vi "Parse Value.vi"(8 "error in (no error)":errorcluster, 11 "Alpaca CLI Parser in":refnum<class "JSON Parser.lvclass">) -> (0 "error out":errorcluster, 2 "Value":variant, 3 "Alpaca CLI Parser out":refnum<class "JSON Parser.lvclass">)   [LabVIEW 2019, in "JKI JSON Serialization.lvlib" / "JSON Parser.lvclass"]
doc: "JKI JSON 1.1.10.37\nTomi Maila - JKI\nCopyright (c) 2017, JKI"
uses:
  JSON Parser.lvclass
  C:/Users/Patrick/Documents/GitHub/Instrument-Framework/lvsrc/SMOs/JSON-RPC-2019/lv-venv/lv.lib/vi.lib/addons/_JKI.lib/Serialization/JSON/Deserializer/Parser/Parser.lvclass
  Parser/Parser.lvclass/Parser.ctl
  JSON Lexer/JSON Token Type.ctl
  Parser/Lookahead.vi
  JSON Lexer/JSON Lexer.lvclass
  JKI JSON Serialization.lvlib
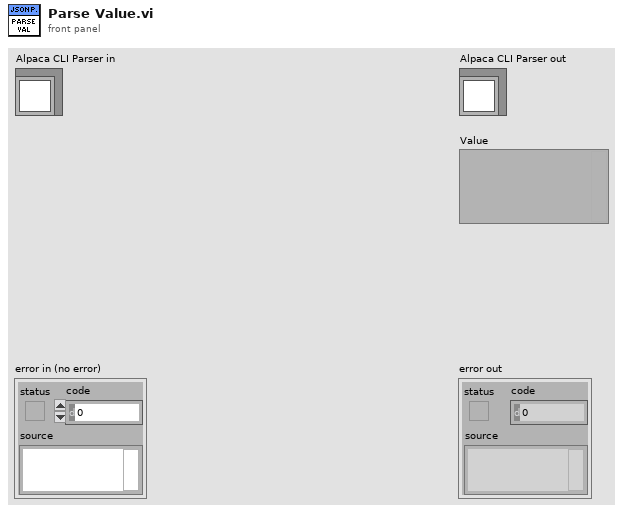
[diagram p1: front panel]
types:
  T1 = typedef "JKI JSON Serialization.lvlib/JSON Lexer.lvclass/JSON Token Type.ctl" = enum32{"unknown", "comma", "end-label", "begin-object", "end-object", "begin-array", "end-array", "quoted-string", "boolean", "exponential-number", "decimal-number", "integer-number", "special-number", "null", "symbol", "whitespace", "EOF"}
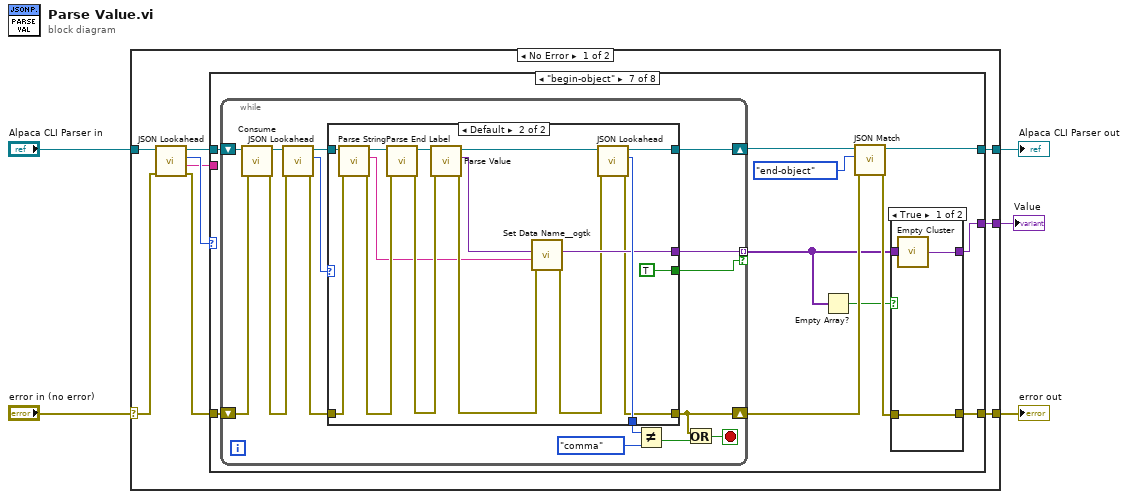
[diagram p0: block diagram]
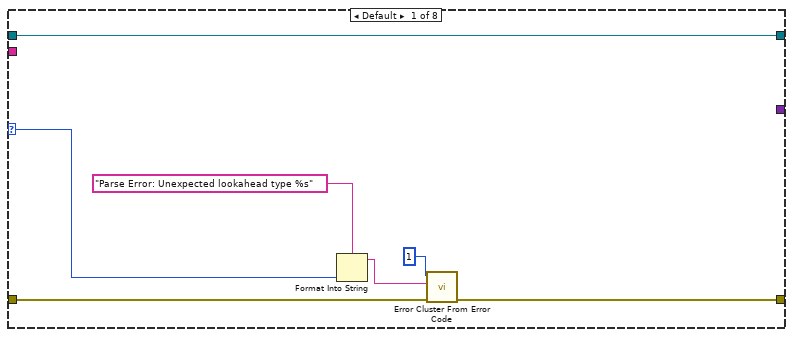
[diagram p2: hidden frame]
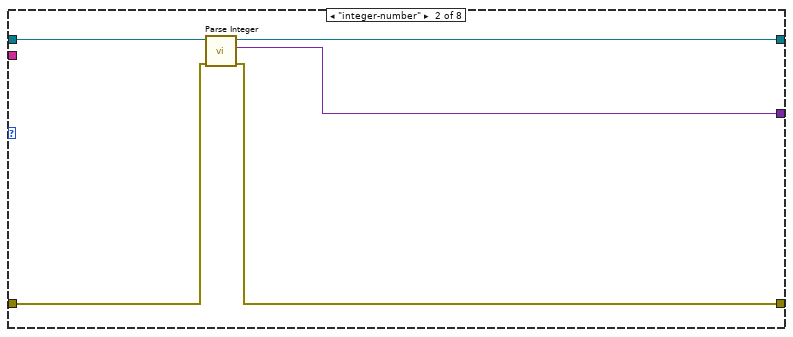
[diagram p3: hidden frame]
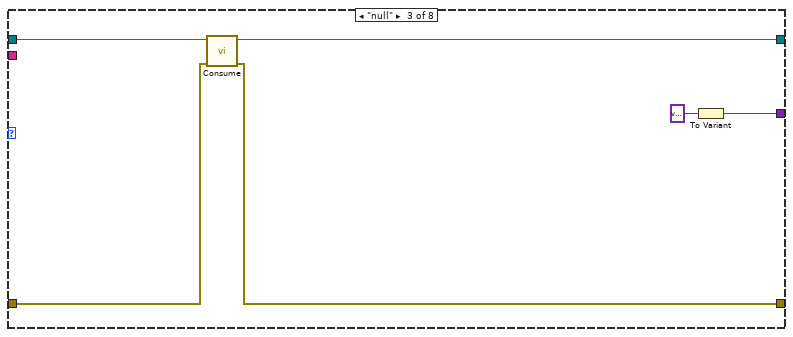
[diagram p4: hidden frame]
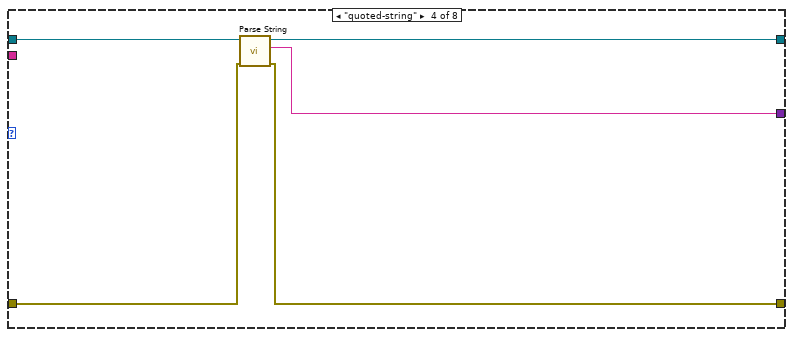
[diagram p5: hidden frame]
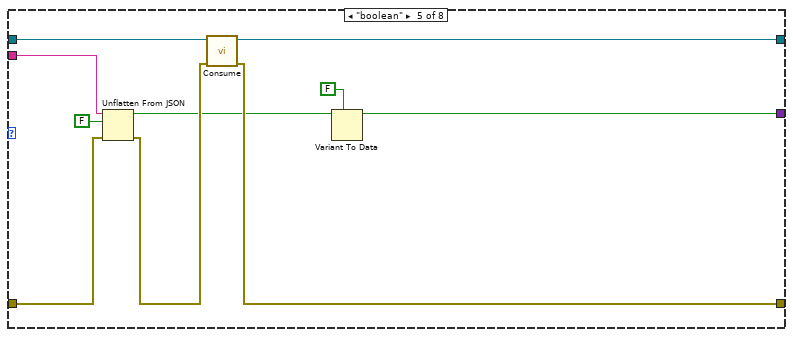
[diagram p6: hidden frame]
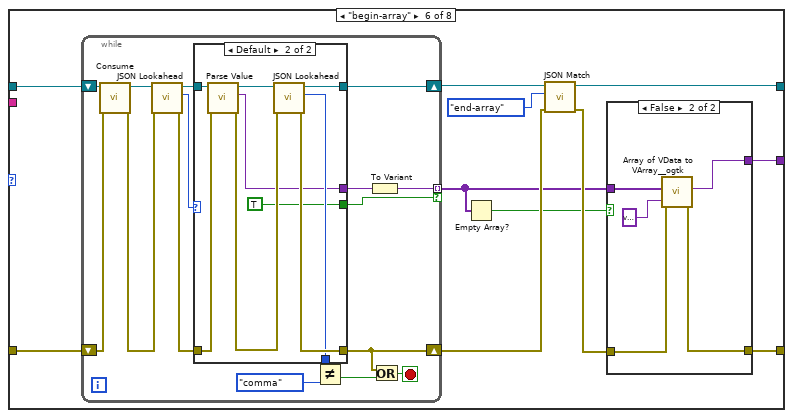
[diagram p7: hidden frame]
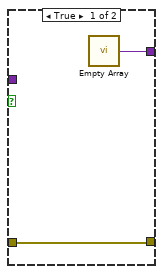
[diagram p8: hidden frame]
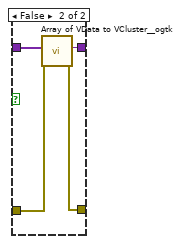
[diagram p10: hidden frame]
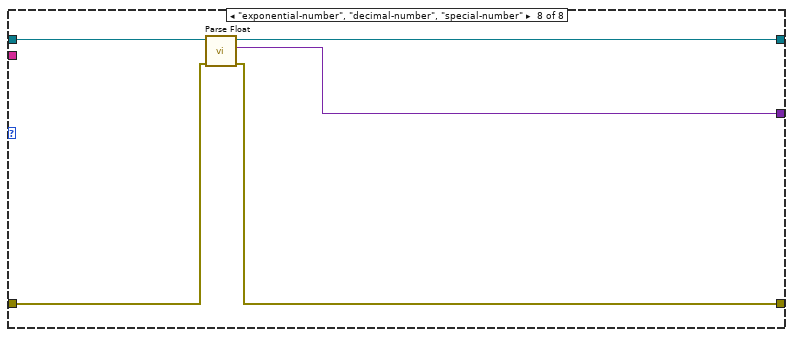
[diagram p12: hidden frame]
diagram:
  n1 = case shown="No Error" "error in (no error)" {
    selector: "error in (no error)" -> [w13 w150]
    tunnel: [w11 w150] -> w4
    tunnel: [w8 w149] -> w2
    tunnel: "Alpaca CLI Parser in" -> [w14 w149]
    tunnel: [w7 _] -> w1
    frame No Error {
      n2 = call "JSON Lookahead.vi"("error in (no error)"=w13, "Alpaca CLI Parser in"=w14) -> ("error out"=w9:errorcluster, "Lookahead Value"=w6:string, "Lookahead Type"=w10:T1, "Alpaca CLI Parser out"=w12:refnum<class "JSON Parser.lvclass">)  [unwired: 6 in]
      n3 = case shown="\"begin-object\"" w10 {
        selector: w10 -> [w17 _ _ _ _ _ _ _]
        tunnel: w12 -> [w15 w26 w32 w37 w47 w58 w104 w148]
        tunnel: [w15 w25 w31 w36 w46 w55 w101 w147] -> w8
        tunnel: [w21 w23 w29 w35 w45 w52 w97 w145] -> w11
        tunnel: w9 -> [w20 w24 w30 w33 w43 w57 w103 w146]
        tunnel: [_ w22 w27 w34 w39 w50 w98 w144] -> w7
        tunnel: w6 -> [_ _ _ _ w44 _ _ _]
        frame Default {
          n4 = Format Into String(format string="Parse Error: Unexpected lookahead type %s" ("error message (\"\")"), w17) -> (resulting string=w16:string)  [unwired: 2 in, 1 out]
          n5 = call <vilib>:"Error Cluster From Error Code.vi"("error in (no error)"=w20, "error message (\"\")"=w16, "error code (0)"=1) -> ("error out"=w21:errorcluster)  [unwired: 6 in]
        }
        frame "integer-number" {
          n6 = call-dynamic "Parse Integer.vi"("error in (no error)"=w24, "Alpaca CLI Parser in"=w26) -> ("error out"=w23:errorcluster, "Value"=w22:variant, "Alpaca CLI Parser out"=w25:refnum<class "JSON Parser.lvclass">)  [unwired: 7 in]
        }
        frame "null" {
          n7 = call-dynamic "Consume.vi"("error in (no error)"=w30, "Alpaca Parser in"=w32) -> ("error out"=w29:errorcluster, "Alpaca Parser out"=w31:refnum<class "JSON Parser.lvclass">)  [unwired: 8 in]
          n8 = To Variant(anything=variant ("Variant")) -> (Variant=w27:variant)
        }
        frame "quoted-string" {
          n9 = call "Parse String.vi"("error in (no error)"=w33, "JSON Parser in"=w37) -> ("error out"=w35:errorcluster, "Parsed String"=w34:string, "JSON Parser out"=w36:refnum<class "JSON Parser.lvclass">)  [unwired: 7 in]
        }
        frame "boolean" {
          n10 = Unflatten From JSON(JSON string=w44, type and defaults=FALSE, error in (no error)=w43) -> (value=w40:bool, error out=w42:errorcluster)  [unwired: 4 in]
          n11 = call-dynamic "Consume.vi"("error in (no error)"=w42, "Alpaca Parser in"=w47) -> ("error out"=w45:errorcluster, "Alpaca Parser out"=w46:refnum<class "JSON Parser.lvclass">)  [unwired: 8 in]
          n12 = Variant To Data(type=FALSE, Variant=w40) -> (data=w39:bool)  [unwired: 1 in, 1 out]
        }
        frame "begin-array" {
          n13 = while {
            shift-right: [w68] -> w54
            shift-left: w57 -> [w80]
            shift-right: [w77] -> w56
            shift-left: w58 -> [w81]
            tunnel: [w67] -> w49 mode=indexing if=w71
            stop <- w70 stop-if-true
            n14 = call-dynamic "Consume.vi"("error in (no error)"=w80, "Alpaca Parser in"=w81) -> ("error out"=w74:errorcluster, "Alpaca Parser out"=w76:refnum<class "JSON Parser.lvclass">)  [unwired: 8 in]
            n15 = call "JSON Lookahead.vi"("error in (no error)"=w74, "Alpaca CLI Parser in"=w76) -> ("error out"=w73:errorcluster, "Lookahead Type"=w72:T1, "Alpaca CLI Parser out"=w75:refnum<class "JSON Parser.lvclass">)  [unwired: 6 in, 1 out]
            n16 = case shown="Default" w72 {
              selector: w72 -> [w82 _]
              tunnel: [w83 w91] -> w68
              tunnel: [w82 w90] -> w78
              tunnel: [w84 w89] -> w77
              tunnel: [_ w88] -> w66
              tunnel: w75 -> [w84 w87]
              tunnel: w73 -> [w83 w86]
              tunnel: [_ TRUE] -> w71
              frame "end-array" {
              }
              frame Default {
                n17 = call-dynamic "Parse Value.vi"("error in (no error)"=w86, "Alpaca CLI Parser in"=w87) -> ("error out"=w92:errorcluster, "Value"=w88:variant, "Alpaca CLI Parser out"=w93:refnum<class "JSON Parser.lvclass">)  [unwired: 7 in]
                n18 = call "JSON Lookahead.vi"("error in (no error)"=w92, "Alpaca CLI Parser in"=w93) -> ("error out"=w91:errorcluster, "Lookahead Type"=w90:T1, "Alpaca CLI Parser out"=w89:refnum<class "JSON Parser.lvclass">)  [unwired: 6 in, 1 out]
              }
            }
            n19 = Not Equal?(x=w78, y=JSON_Token_Type."comma" ("Lookahead Type")) -> (x != y?=w69:bool)
            n20 = To Variant(anything=w66) -> (Variant=w67:variant)
            n21 = Or(x=w68, y=w69) -> (x .or. y?=w70:bool)
          }
          n22 = Empty Array?(array=w49) -> (empty?=w48:bool)
          n23 = call "JSON Match.vi"("error in (no error)"=w54, "JSON Token"=JSON_Token_Type."end-array" ("Lookahead Type"), "Alpaca CLI Parser in"=w56) -> ("error out"=w51:errorcluster, "Alpaca CLI Parser out"=w55:refnum<class "JSON Parser.lvclass">)  [unwired: 7 in]
          n24 = case shown="False" w48 {
            tunnel: [w60 w65] -> w52
            tunnel: w51 -> [w60 w64]
            tunnel: [w59 w63] -> w50
            tunnel: w49 -> [_ w61]
            frame True {
              n25 = call "Empty Array.vi"() -> ("Empty Cluster"=w59:variant)
            }
            frame False {
              n26 = call "Array of VData to VArray__ogtk.vi"("error in (no error)"=w64, "Element Type (when empty)"=variant, "1D Array of VData"=w61) -> ("error out"=w65:errorcluster, "VArray"=w63:variant)  [unwired: 7 in]
            }
          }
        }
        frame "begin-object" {
          n27 = while {
            shift-right: [w117] -> w100
            shift-left: w103 -> [w124]
            shift-right: [w121] -> w102
            shift-left: w104 -> [w125]
            tunnel: [w120] -> w94 mode=indexing if=w111
            stop <- w119 stop-if-true
            n28 = call-dynamic "Consume.vi"("error in (no error)"=w124, "Alpaca Parser in"=w125) -> ("error out"=w114:errorcluster, "Alpaca Parser out"=w116:refnum<class "JSON Parser.lvclass">)  [unwired: 8 in]
            n29 = call "JSON Lookahead.vi"("error in (no error)"=w114, "Alpaca CLI Parser in"=w116) -> ("error out"=w113:errorcluster, "Lookahead Type"=w112:T1, "Alpaca CLI Parser out"=w115:refnum<class "JSON Parser.lvclass">)  [unwired: 6 in, 1 out]
            n30 = case shown="Default" w112 {
              tunnel: [_ w143] -> w122
              tunnel: [w127 w142] -> w121
              tunnel: [_ w141] -> w120
              tunnel: [w126 w140] -> w117
              tunnel: w115 -> [w127 w131]
              tunnel: w113 -> [w126 w130]
              tunnel: [_ TRUE] -> w111
              frame "end-object" {
              }
              frame Default {
                n31 = call "Parse String.vi"("error in (no error)"=w130, "JSON Parser in"=w131) -> ("error out"=w136:errorcluster, "Parsed String"=w132:string, "JSON Parser out"=w138:refnum<class "JSON Parser.lvclass">)  [unwired: 7 in]
                n32 = call-dynamic "Parse End Label.vi"("error in (no error)"=w136, "Alpaca CLI Parser in"=w138) -> ("error out"=w135:errorcluster, "Alpaca CLI Parser out"=w137:refnum<class "JSON Parser.lvclass">)  [unwired: 8 in]
                n33 = call-dynamic "Parse Value.vi"("error in (no error)"=w135, "Alpaca CLI Parser in"=w137) -> ("error out"=w134:errorcluster, "Value"=w128:variant, "Alpaca CLI Parser out"=w139:refnum<class "JSON Parser.lvclass">)  [unwired: 7 in]
                n34 = call "Set Data Name__ogtk.vi"("error in (no error)"=w134, "Data Name"=w132, "Data"=w128) -> ("error out"=w133:errorcluster, "Renamed Data"=w141:variant)  [unwired: 7 in]
                n35 = call "JSON Lookahead.vi"("error in (no error)"=w133, "Alpaca CLI Parser in"=w139) -> ("error out"=w140:errorcluster, "Lookahead Type"=w143:T1, "Alpaca CLI Parser out"=w142:refnum<class "JSON Parser.lvclass">)  [unwired: 6 in, 1 out]
              }
            }
            n36 = Not Equal?(x=w122, y=JSON_Token_Type."comma" ("Lookahead Type")) -> (x != y?=w118:bool)
            n37 = Or(x=w117, y=w118) -> (x .or. y?=w119:bool)
          }
          n38 = Empty Array?(array=w94) -> (empty?=w95:bool)
          n39 = call "JSON Match.vi"("error in (no error)"=w100, "JSON Token"=JSON_Token_Type."end-object" ("Lookahead Type"), "Alpaca CLI Parser in"=w102) -> ("error out"=w96:errorcluster, "Alpaca CLI Parser out"=w101:refnum<class "JSON Parser.lvclass">)  [unwired: 7 in]
          n40 = case shown="True" w95 {
            tunnel: [w105 w110] -> w98
            tunnel: [w106 w109] -> w97
            tunnel: w96 -> [w106 w108]
            tunnel: w94 -> [_ w107]
            frame True {
              n41 = call "Empty Cluster.vi"() -> ("Empty Cluster"=w105:variant)
            }
            frame False {
              n42 = call "Array of VData to VCluster__ogtk.vi"("error in (no error)"=w108, "Array"=w107) -> ("error out"=w109:errorcluster, "VCluster"=w110:variant)  [unwired: 8 in]
            }
          }
        }
        frame "exponential-number", "decimal-number", "special-number" {
          n43 = call-dynamic "Parse Float.vi"("error in (no error)"=w146, "Alpaca CLI Parser in"=w148) -> ("error out"=w145:errorcluster, "Value"=w144:variant, "Alpaca CLI Parser out"=w147:refnum<class "JSON Parser.lvclass">)  [unwired: 7 in]
        }
      }
    }
    frame Error {
    }
  }
  "error out" <- w4
  "Alpaca CLI Parser out" <- w2
  "Value" <- w1
